vi "Control_tb.vi"() -> ()   [LabVIEW 2018]
panel:
  out "Execution:State":T1(ring)
  out "Is Instance":bool
  out "Is Running Interactively":bool
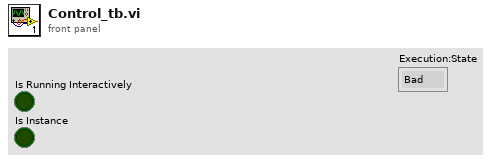
[diagram p1: front panel]
types:
  T1 = enum32{"Bad", "Idle", "Run top level", "Running"}
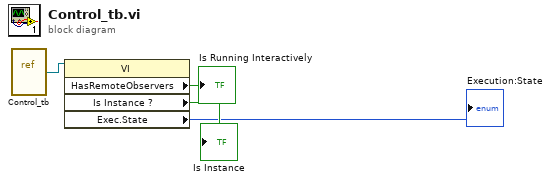
[diagram p0: block diagram]
diagram:
  n1 = vi-ref "Control_tb.vi"() -> (w4:refnum<vi>)
  n2 = property class="VI"(reference=w4) -> ("HasRemoteObservers"=→"Is Running Interactively":bool, "Is Instance ?"=→"Is Instance":bool, "Exec.State"=→"Execution:State":T1)  [unwired: 1 in, 2 out]
